vi "Get Name.vi"(11 "IProvide Configurations in":refnum<class "IProvide Configurations.lvclass">) -> (2 "Name":string, 3 "IProvide Configurations out":refnum<class "IProvide Configurations.lvclass">)   [LabVIEW 2023, in "IProvide Configurations.lvclass"]
uses:
  IProvide Configurations.lvclass
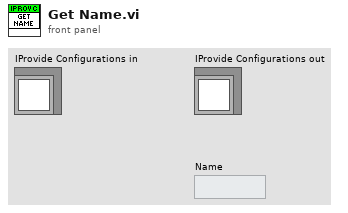
[diagram p1: front panel]
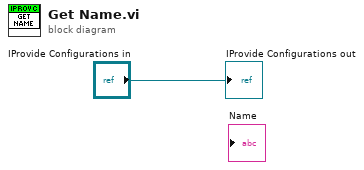
[diagram p0: block diagram]
diagram:
  "IProvide Configurations out" <- "IProvide Configurations in"
